vi "Find next tabbable element.vi"(9 "Start column (0)":i32, 10 "Start row (0)":i32, 11 "DataElements":refnum<class "DatagridElement.lvclass">[][](array[class])) -> (1 "Next element column":i32, 2 "Next element row":i32)   [LabVIEW 2018, in "D Datagrid Library.lvlib" / "D_Datagrid.lvclass"]
uses:
  D_Datagrid.lvclass
  DatagridElement/DatagridElement.lvclass
  DatagridElement/DatagridElement.lvclass/DatagridElement.ctl
  DatagridElement/Read Enabled state.vi
panel:
  out "Found?":bool
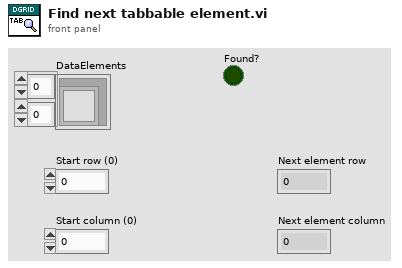
[diagram p1: front panel]
types:
  T1 = enum8{"Enabled", "Disabled", "Disabled and Grayed Out"}
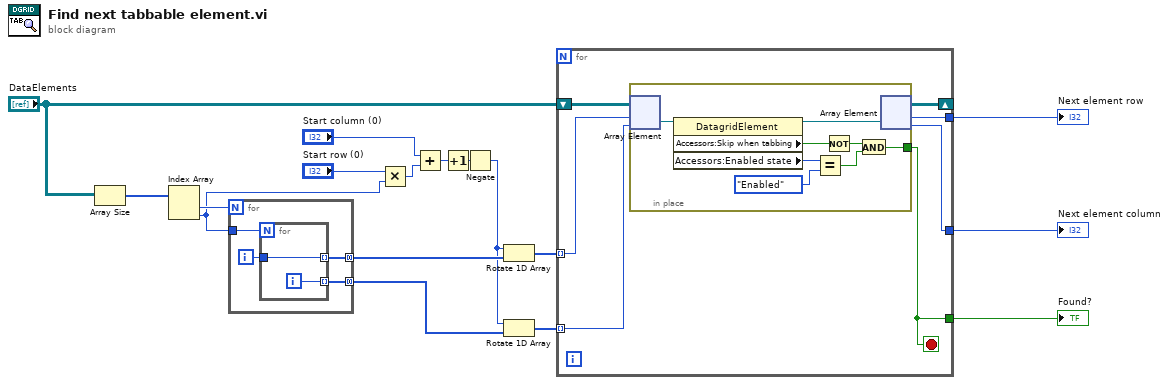
[diagram p0: block diagram]
diagram:
  n1 = Array Size(array="DataElements") -> (size(s)=w11:i32[])
  n2 = Index Array(array=w11) -> (element #1=w15:i32, element #2=w7:i32)  [unwired: 2 in]
  n3 = for {
    N: w15 -> [_]
    tunnel: w7 -> [w21]
    tunnel: [w20] -> w8 mode=concatenating
    tunnel: [w18] -> w9 mode=concatenating
    i -> [w19]
    n4 = for {
      N: w21 -> [_]
      tunnel: [w23] -> w20 mode=indexing
      tunnel: [w22] -> w18 mode=indexing
      tunnel: w19 -> [w22]
      i -> [w23]
    }
  }
  n5 = Multiply(x="Start row (0)", y=w7) -> (x*y=w5:i32)
  n6 = Add(x="Start column (0)", y=w5) -> (x+y=w3:i32)
  n7 = Increment(x=w3) -> (x+1=w2:i32)
  n8 = Negate(x=w2) -> (-x=w1:i32)
  n9 = Rotate 1D Array(1:w9, 2:w1) -> (0:w10:i32[])
  n10 = Rotate 1D Array(1:w8, 2:w1) -> (0:w14:i32[])
  n11 = for {
    shift-right: [w29] -> _
    shift-left: "DataElements" -> [w30]
    tunnel: [w28] -> w16
    tunnel: w10 -> [w27] mode=indexing
    tunnel: w14 -> [w26] mode=indexing
    tunnel: [w25] -> w13
    tunnel: [w24] -> w12
    stop <- w28 stop-if-true
    n12 = in-place {
      in-place-border: [w31] -> w28
      n13 = in-place-array #1(w30, w27, w26) -> (w38:refnum<class "DatagridElement.lvclass">)
      n14 = property class="DatagridElement"(reference=w38) -> (reference out=w37:refnum<class "DatagridElement.lvclass">, "Accessors:Skip when tabbing"=w34:bool, "Accessors:Enabled state"=w36:T1)  [unwired: 1 in, 1 out]
      n15 = Equal?(x=w36, y=T1."Enabled") -> (x = y?=w32:bool)
      n16 = Not(x=w34) -> (.not. x?=w33:bool)
      n17 = And(x=w33, y=w32) -> (x .and. y?=w31:bool)
      n18 = in-place-array #1(w37) -> (w29:refnum<class "DatagridElement.lvclass">[][], w25:i32, w24:i32)
    }
  }
  "Next element row" <- w13
  "Next element column" <- w12
  "Found?" <- w16
